vi "CAN BL Write.vi"(4 "TimeOut":u32, 5 "DataNum":u32, 6 "pData":u8[](array[numeric])=array[20480 elements], 7 "AddrOffset":u32, 9 "NodeAddr":u16, 10 "CANIndex":i32, 11 "DevIndex":i32) -> (3 "function return":i32)   [LabVIEW 2010, in "usb2can.lvlib"]
doc: "int WINAPI CAN_BL_Write(int DevIndex,int CANIndex,unsigned short NodeAddr,unsigned int AddrOffset,unsigned char *pData,unsigned int DataNum,unsigned int TimeOut);"
uses:
  usb2can.lvlib
  USB2XXX.dll
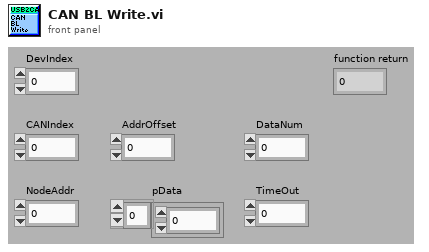
[diagram p1: front panel]
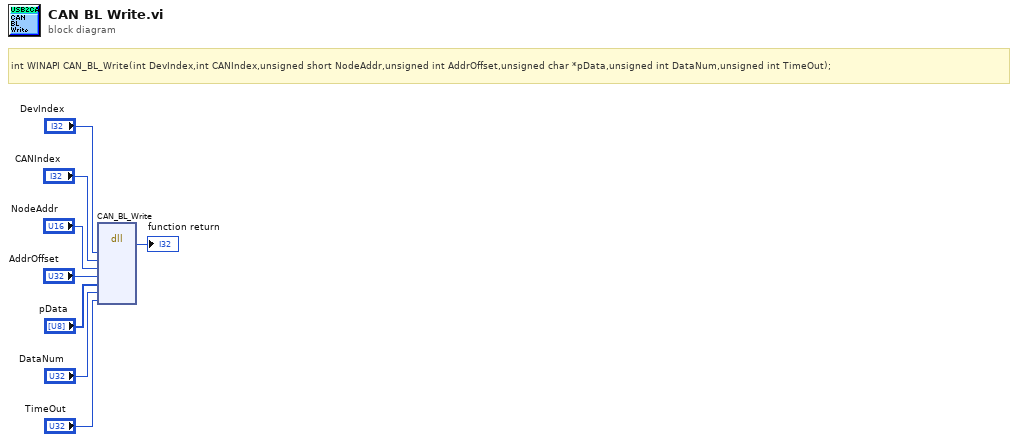
[diagram p0: block diagram]
diagram:
  # "int WINAPI CAN_BL_Write(int DevIndex,int CANIndex,unsigned short NodeAddr,unsigned int AddrOffset,unsigned char *pData,unsigned int DataNum,unsigned int TimeOut);"
  n1 = dll-call lib="F:/OtherWork/STM32/CAN-Bootloader/software/CANBootloader-Labview/usb2can/USB2XXX.*" fn="CAN_BL_Write"("DevIndex"="DevIndex", "CANIndex"="CANIndex", "NodeAddr"="NodeAddr", "AddrOffset"="AddrOffset", "pData"="pData", "DataNum"="DataNum", "TimeOut"="TimeOut") -> ("return type"=→"function return":i32)  [unwired: 10 in, 2 out]
